vi "D2SParser - Private - Function - Read Character Strength.vi"(8 "error in (no error)":errorcluster, 9 "Present?":bool, 10 "Position":i64, 11 "D2SParser in":refnum<class "D2SParser.lvclass">) -> (0 "error out":errorcluster, 3 "D2SParser out":refnum<class "D2SParser.lvclass">)   [LabVIEW 2015, in "D2SParser.lvclass"]
uses:
  D2SParser.lvclass
  D2SParser.lvclass/D2SParser.ctl
  D2Character/D2Character.lvclass/D2Character.ctl
  D2Character/D2Character - Accessors - Set Strength.vi
  D2SParser - Private - Helper - Read Long.vi
  D2Character/D2Character.lvclass
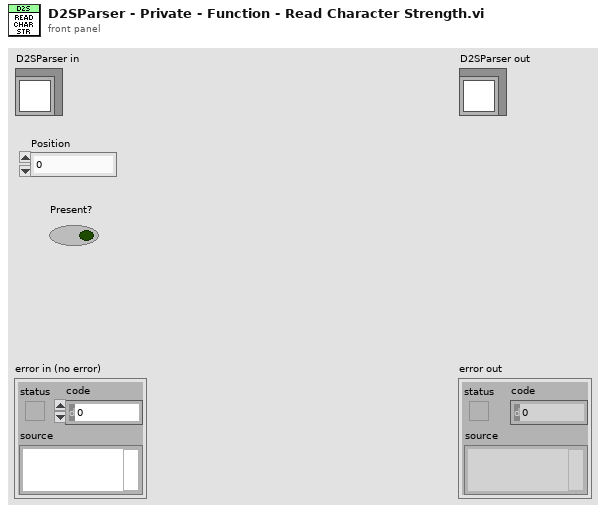
[diagram p1: front panel]
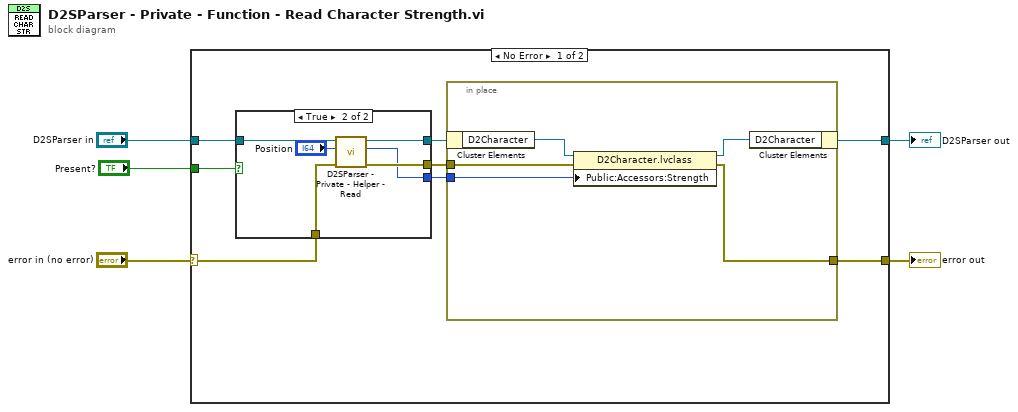
[diagram p0: block diagram]
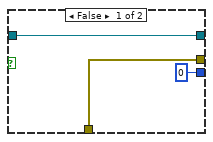
[diagram p2: hidden frame]
diagram:
  n1 = case shown="No Error" "error in (no error)" {
    selector: "error in (no error)" -> [w12 w29]
    tunnel: [w9 w29] -> w4
    tunnel: [w8 w28] -> w2
    tunnel: "D2SParser in" -> [w13 w28]
    tunnel: "Present?" -> [w6 _]
    frame No Error {
      n2 = case shown="True" w6 {
        tunnel: w13 -> [w16 w22]
        tunnel: w12 -> [w14 w21]
        tunnel: [w16 w20] -> w11
        tunnel: [w14 w19] -> w10
        tunnel: [u32 0 ("long") w17] -> w7
        frame False {
        }
        frame True {
          n3 = call-poly "D2SParser - Private - Helper - Read.vi"("error in (no error)"=w21, "Position"="Position", "D2SParser in"=w22) -> ("error out"=w19:errorcluster, "long"=w17:u32, "D2SParser out"=w20:refnum<class "D2SParser.lvclass">)  [unwired: 6 in]
        }
      }
      n4 = in-place {
        in-place-border: w10 -> [w25]
        in-place-border: [w24] -> w9
        in-place-border: w7 -> [w23]
        n5 = in-place-cluster #1(w11) -> ("D2Character"=w27:refnum<class "D2Character.lvclass">)
        n6 = property class="D2Character.lvclass"(reference=w27, error in=w25, "Public:Accessors:Strength"=w23) -> (reference out=w26:refnum<class "D2Character.lvclass">, error out=w24:errorcluster)
        n7 = in-place-cluster #1("D2Character"=w26) -> (w8:refnum<class "D2SParser.lvclass">)
      }
    }
    frame Error {
    }
  }
  "error out" <- w4
  "D2SParser out" <- w2
